vi "set output range.vi"(9 "output range low (requested)":dbl, 10 "output range high (requested)":dbl, 11 "Data Value Reference in":refnum<data-value>) -> (0 "error out":errorcluster, 1 "output range low (real)":dbl, 2 "output range high (real)":dbl)   [LabVIEW 2013, in "My Awesome Control Modules editor node.lvclass"]
uses:
  My Awesome Control Modules editor node.lvclass
  <vilib>/NI/Tag Bus Data Framework/control module/configuration/control module configuration.lvclass
  <vilib>/NI/Tag Bus/tag/tag descriptor.lvclass
  <vilib>/NI/Tag Bus/tag/default value polymorphs/write default value Double.vi
  <vilib>/NI/Tag Bus Data Framework/control module/editor node/control module editor.lvclass
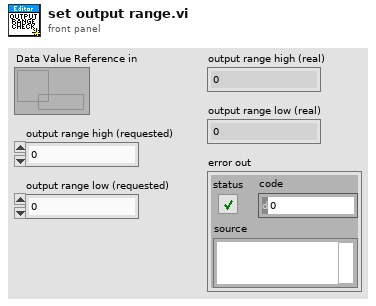
[diagram p1: front panel]
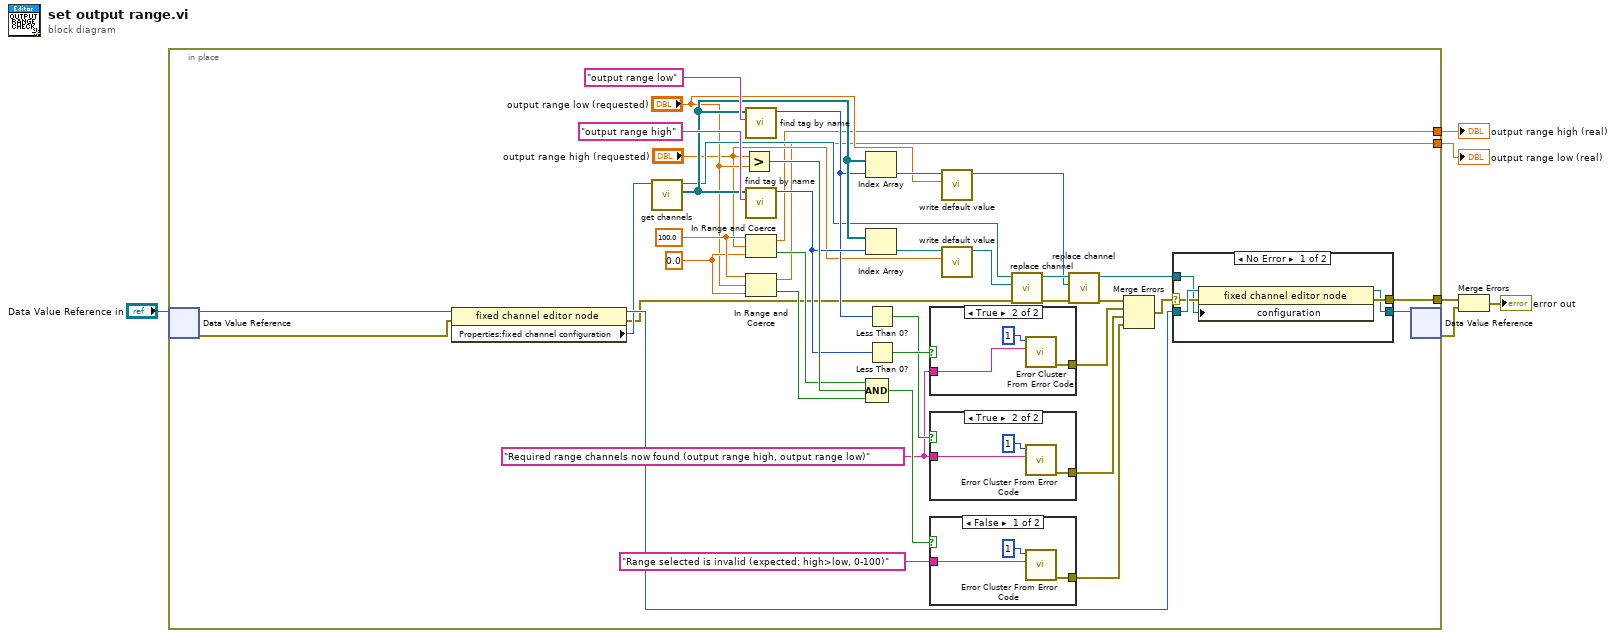
[diagram p0: block diagram]
diagram:
  n1 = in-place {
    in-place-border: [w42] -> w4
    in-place-border: [w8] -> w2
    in-place-border: [w7] -> w1
    w25 = "Required range channels now found (output range high, output range low)" ("error message (\"\")")
    w33 = 100.0 ("upper limit")
    w32 = 0.0 ("lower limit")
    n2 = in-place-dvr #1("Data Value Reference in") -> (w45:refnum<class "control module editor.lvclass">, w44:errorcluster)
    n3 = property class="fixed channel editor node"(reference=w45, error in=w44) -> (reference out=w43:refnum<class "control module editor.lvclass">, error out=w17:errorcluster, "Properties:fixed channel configuration"=w40:refnum<class "control module configuration.lvclass">)
    n4 = call-dynamic "get channels.vi"("fixed channel configuration in"=w40) -> ("channels"=w37:refnum<class "TBM channel.lvclass">[], "fixed channel configuration out"=w16:refnum<class "control module configuration.lvclass">)  [unwired: 9 in]
    n5 = Greater?(x="output range high (requested)", y="output range low (requested)") -> (0:w36:bool)
    n6 = call <vilib>:"find tag by name.vi"("name"="output range low" ("String"), "tags in"=w37) -> ("index"=w28:i32)  [unwired: 9 in]
    n7 = call <vilib>:"find tag by name.vi"("name"="output range high" ("String"), "tags in"=w37) -> ("index"=w29:i32)  [unwired: 9 in]
    n8 = In Range and Coerce(upper limit=w33, x="output range high (requested)", lower limit=w32) -> (coerced(x)=w8:dbl, In Range?=w35:bool)
    n9 = In Range and Coerce(upper limit=w33, x="output range low (requested)", lower limit=w32) -> (coerced(x)=w7:dbl, In Range?=w34:bool)
    n10 = Index Array(array=w37, index=w28) -> (element=w12:refnum<class "TBM channel.lvclass">)
    n11 = Index Array(array=w37, index=w29) -> (element=w14:refnum<class "TBM channel.lvclass">)
    n12 = Compound Arithmetic op=AND(w35, w36, w34) -> (w31:bool)
    n13 = Less Than 0?(x=w28) -> (x < 0?=w26:bool)
    n14 = Less Than 0?(x=w29) -> (x < 0?=w27:bool)
    n15 = case shown="True" w27 {
      tunnel: w25 -> [_ w50]
      tunnel: [_ w49] -> w21
      frame False {
      }
      frame True {
        n16 = call <vilib>:"Error Cluster From Error Code.vi"("error message (\"\")"=w50, "error code (0)"=1) -> ("error out"=w49:errorcluster)  [unwired: 7 in]
      }
    }
    n17 = case shown="True" w26 {
      tunnel: w25 -> [_ w47]
      tunnel: [_ w46] -> w22
      frame False {
      }
      frame True {
        n18 = call <vilib>:"Error Cluster From Error Code.vi"("error message (\"\")"=w47, "error code (0)"=1) -> ("error out"=w46:errorcluster)  [unwired: 7 in]
      }
    }
    n19 = case shown="False" w31 {
      tunnel: "Range selected is invalid (expected: high>low, 0-100)" ("error message (\"\")") -> [w53 _]
      tunnel: [w52 _] -> w23
      frame False {
        n20 = call <vilib>:"Error Cluster From Error Code.vi"("error message (\"\")"=w53, "error code (0)"=1) -> ("error out"=w52:errorcluster)  [unwired: 7 in]
      }
      frame True {
      }
    }
    n21 = call-poly <vilib>:"write default value.vi"("default value"="output range low (requested)", "system tag in"=w12) -> ("system tag out"=w11:refnum<class "TBM channel.lvclass">)  [unwired: 8 in, 1 out]
    n22 = call-poly <vilib>:"write default value.vi"("default value"="output range high (requested)", "system tag in"=w14) -> ("system tag out"=w13:refnum<class "TBM channel.lvclass">)  [unwired: 8 in, 1 out]
    n23 = call <vilib>:"replace channel.vi"("error in"=w17, "channel"=w13, "fixed module parent implementation configuration in"=w16) -> ("error out"=w18:errorcluster, "fixed module parent implementation configuration out"=w15:refnum<class "control module configuration.lvclass">)  [unwired: 7 in]
    n24 = call <vilib>:"replace channel.vi"("error in"=w18, "channel"=w11, "fixed module parent implementation configuration in"=w15) -> ("error out"=w20:errorcluster, "fixed module parent implementation configuration out"=w19:refnum<class "control module configuration.lvclass">)  [unwired: 7 in]
    n25 = Merge Errors(w20, w21, w22, w23) -> (w24:errorcluster)
    n26 = case shown="No Error" w24 {
      selector: w24 -> [w58 w61]
      tunnel: w43 -> [w59 w60]
      tunnel: [w57 w61] -> w42
      tunnel: [w56 w60] -> w41
      tunnel: w19 -> [w55 _]
      frame No Error {
        n27 = property class="fixed channel editor node"(reference=w59, error in=w58, "configuration"=w55) -> (reference out=w56:refnum<class "control module editor.lvclass">, error out=w57:errorcluster)
      }
      frame Error {
      }
    }
    n28 = in-place-dvr #1(w41) -> (w5:errorcluster)  [unwired: 1 out]
  }
  "output range high (real)" <- w2
  "output range low (real)" <- w1
  n29 = Merge Errors(w4, w5) -> (→"error out":errorcluster)
